vi "IR GALVO CONTROL (SINGLE SPOT).vi"() -> ()   [LabVIEW 2017]
uses:
  <vilib>/DAQmx/write.llb/DAQmx Write (Analog 1D DBL NChan 1Samp).vi
  <vilib>/DAQmx/configure/timing.llb/DAQmx Timing (Sample Clock).vi
  <vilib>/Utility/file.llb/Read Delimited Spreadsheet (DBL).vi
  <vilib>/DAQmx/miscellaneous.llb/DAQmx Fill In Error Info.vi
panel:
  in  "Calibrated":bool
  in  "X":i32
  in  "Y":i32
  in  "GALVO Input Voltage (V)":T1={"GALVO 1"={"X"=-1.0, "Y "=1.0}, "GALVO 2"={"X"=0.0, "Y "=0.0}, "GALVO 3"={"X"=0.0, "Y "=0.0}, "GALVO 4"={"X"=0.0, "Y "=0.0}} {"GALVO 4"."Y" format="%.3f"; "GALVO 4"."X" format="%.3f"; "GALVO 3"."Y" format="%.3f"; "GALVO 3"."X" format="%.3f"; "GALVO 2"."Y" format="%.3f"; "GALVO 2"."X" format="%.3f"; "GALVO 1"."Y" format="%.3f"; "GALVO 1"."X" format="%.3f"}
  in  "Stop Button":bool
  in  "DAQmx Task Name":refnum<k21>="GALVO"
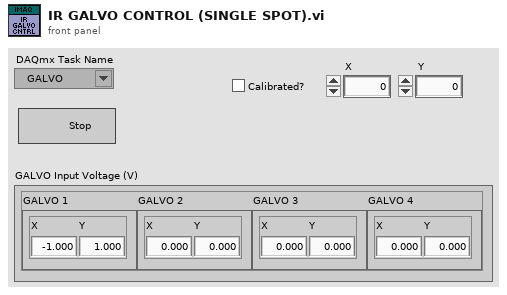
[diagram p1: front panel]
types:
  T1 = cluster{"GALVO 1":cluster{"X":dbl, "Y ":dbl}, "GALVO 2":cluster{"X":dbl, "Y ":dbl}, "GALVO 3":cluster{"X":dbl, "Y ":dbl}, "GALVO 4":cluster{"X":dbl, "Y ":dbl}}
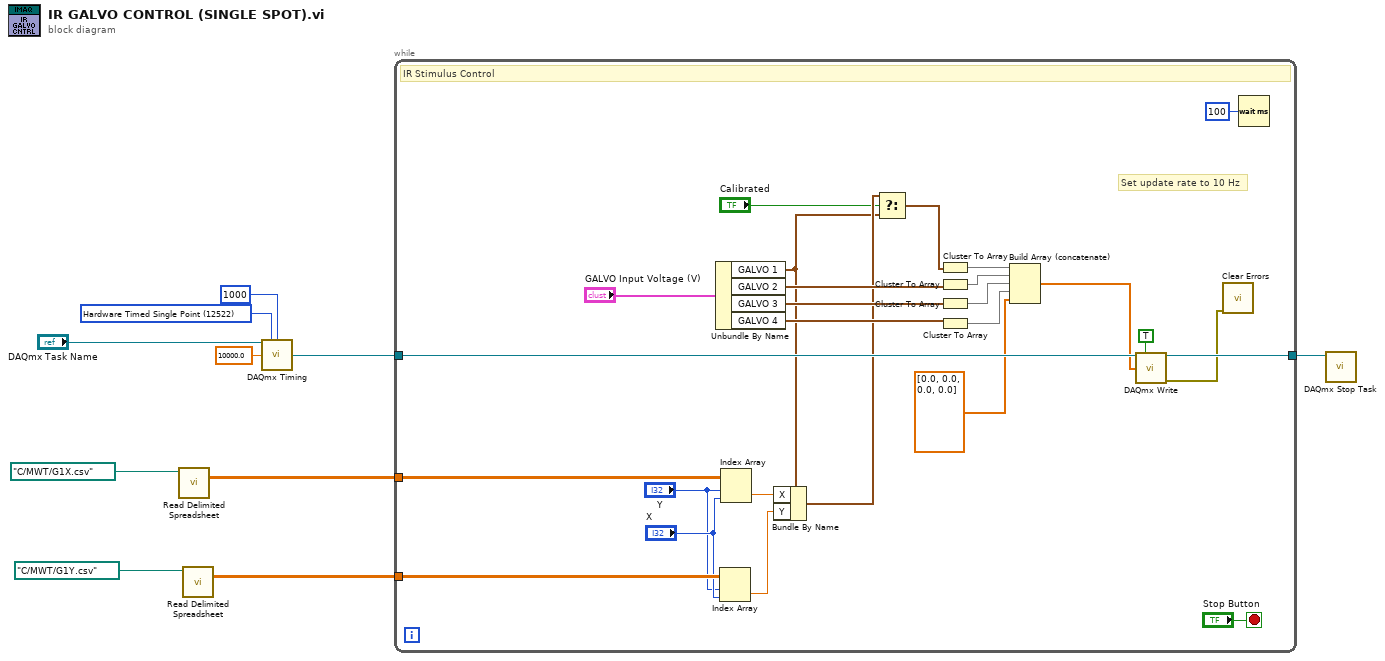
[diagram p0: block diagram]
diagram:
  w7 = 12522 items=["Finite Samples"=10178, "Continuous Samples"=10123, "Hardware Timed Single Point"=12522] ("sample mode")
  n1 = call-poly <vilib>:"Read Delimited Spreadsheet.vi"("file path (dialog if empty)"=path "C:/MWT/G1X.csv") -> ("all rows"=w2:dbl[][])  [unwired: 9 in, 5 out]
  n2 = call-poly <vilib>:"Read Delimited Spreadsheet.vi"("file path (dialog if empty)"=path "C:/MWT/G1Y.csv") -> ("all rows"=w1:dbl[][])  [unwired: 9 in, 5 out]
  n3 = call-poly <vilib>:"DAQmx Timing.vi"("task/channels in"="DAQmx Task Name", "sample mode"=w7, "samples per channel"=1000, "rate"=10000.0) -> ("task out"=w8:refnum<k21>)  [unwired: 10 in, 1 out]
  n4 = while {
    tunnel: [w36] -> w10
    tunnel: w8 -> [w23]
    tunnel: w2 -> [w21]
    tunnel: w1 -> [w20]
    stop <- "Stop Button" stop-if-true
    # "Set update rate to 10 Hz"
    # "IR Stimulus Control"
    n5 = Unbundle By Name("GALVO Input Voltage (V)") -> ("GALVO 1"=w13:cluster{"X":dbl, "Y ":dbl}, "GALVO 2"=w30:cluster{"X":dbl, "Y ":dbl}, "GALVO 3"=w29:cluster{"X":dbl, "Y ":dbl}, "GALVO 4"=w28:cluster{"X":dbl, "Y ":dbl})
    n6 = Index Array(array=w20, index (row)="Y", index (col)="X") -> (element=w16:dbl)
    n7 = Index Array(array=w21, index (row)="Y", index (col)="X") -> (element=w17:dbl)
    n8 = Bundle By Name(cluster=w13, "X"=w17, "Y"=w16) -> (w15:cluster{"X":dbl, "Y ":dbl})
    n9 = Select(t=w15, s="Calibrated", f=w13) -> (s? t:f=w14:cluster{"X":dbl, "Y ":dbl})
    n10 = Cluster To Array(cluster=w14) -> (array=w27:dbl[])
    n11 = Cluster To Array(cluster=w30) -> (array=w26:dbl[])
    n12 = Cluster To Array(cluster=w29) -> (array=w25:dbl[])
    n13 = Cluster To Array(cluster=w28) -> (array=w24:dbl[])
    n14 = Build Array (concatenate)(w27, w26, w25, w24, dbl[] [0.0, 0.0, 0.0, 0.0] ("array")) -> (w22:dbl[])
    n15 = call-poly <vilib>:"DAQmx Write.vi"("task/channels in"=w23, "auto start"=TRUE, "data"=w22) -> ("task out"=w36:refnum<k21>, "error out"=w32:errorcluster)  [unwired: 10 in, 1 out]
    n16 = call <vilib>:"Clear Errors.vi"("error in (no error)"=w32) -> ()  [unwired: 5 in, 2 out]
    n17 = Wait (ms)(milliseconds to wait=u32 100) -> ()  [unwired: 1 out]
  }
  n18 = call <vilib>:"DAQmx Stop Task.vi"("task/channels in"=w10) -> ()  [unwired: 13 in, 2 out]
